vi "Master_DAQ_ReadVIN.vi"() -> (0 "cRIO Data":T1)   [LabVIEW 2017]
uses:
  TypeDef_cRIOData.ctl
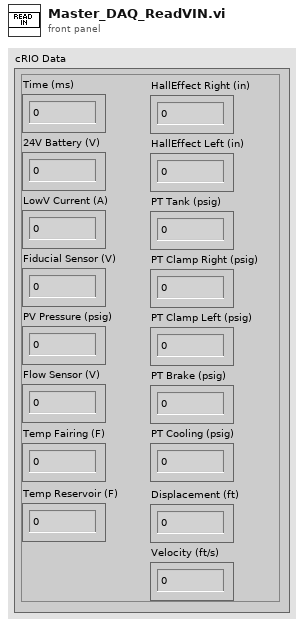
[diagram p1: front panel]
types:
  T1 = typedef "TypeDef_cRIOData.ctl" = cluster{"Time (ms)":dbl, "24V Battery (V)":dbl, "LowV Current (A)":dbl, "Fiducial Sensor (V)":dbl, "PV Pressure (psig)":dbl, "Flow Sensor (V)":dbl, "Temp Fairing (F)":dbl, "Temp Reservoir (F)":dbl, "HallEffect Right (in)":dbl, "HallEffect Left (in)":dbl, "PT Tank (psig)":dbl, "PT Clamp Right (psig)":dbl, "PT Clamp Left (psig)":dbl, "PT Brake (psig)":dbl, "PT Cooling (psig)":dbl, "Displacement (ft)":dbl, "Velocity (ft/s)":dbl}
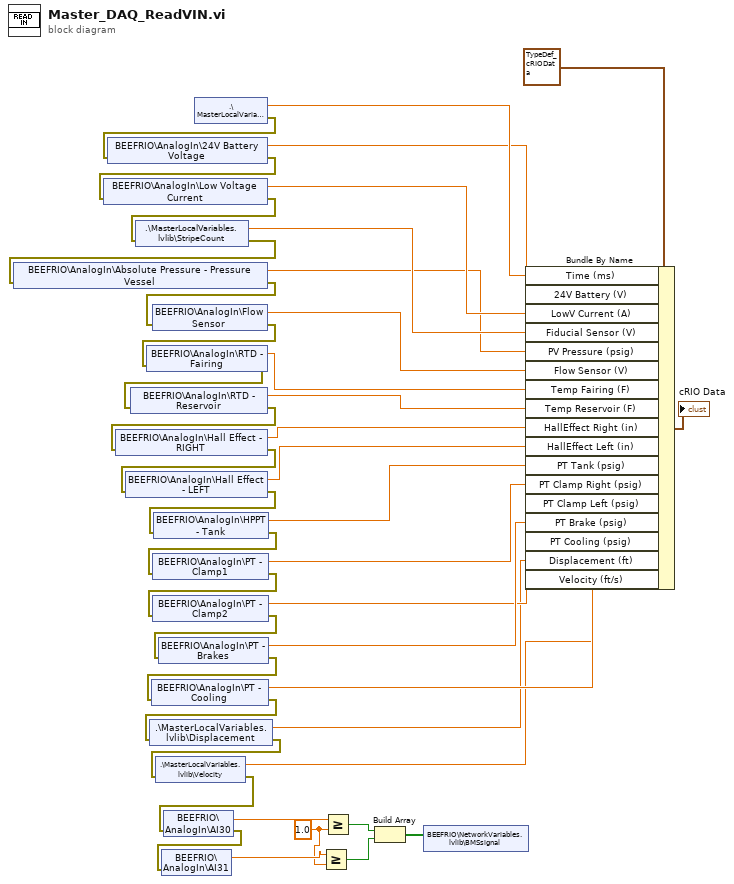
[diagram p0: block diagram]
diagram:
  w4 = 1.0 ("y")
  n1 = shared-variable ".\\MasterLocalVariables.lvlib\\Time"() -> (w41:dbl, error out=w40:errorcluster)  [unwired: 1 in]
  n2 = shared-variable "BEEFRIO\\AnalogIn\\24V Battery Voltage"(error in=w40) -> (w26:dbl, error out=w39:errorcluster)
  n3 = shared-variable "BEEFRIO\\AnalogIn\\Low Voltage Current"(error in=w39) -> (w25:dbl, error out=w38:errorcluster)
  n4 = shared-variable ".\\MasterLocalVariables.lvlib\\StripeCount"(error in=w38) -> (w24:dbl, error out=w37:errorcluster)
  n5 = shared-variable "BEEFRIO\\AnalogIn\\Absolute Pressure - Pressure Vessel"(error in=w37) -> (w23:dbl, error out=w36:errorcluster)
  n6 = shared-variable "BEEFRIO\\AnalogIn\\Flow Sensor"(error in=w36) -> (w22:dbl, error out=w35:errorcluster)
  n7 = shared-variable "BEEFRIO\\AnalogIn\\RTD - Fairing"(error in=w35) -> (w21:dbl, error out=w34:errorcluster)
  n8 = shared-variable "BEEFRIO\\AnalogIn\\RTD - Reservoir"(error in=w34) -> (w20:dbl, error out=w33:errorcluster)
  n9 = shared-variable "BEEFRIO\\AnalogIn\\Hall Effect - RIGHT"(error in=w33) -> (w19:dbl, error out=w32:errorcluster)
  n10 = shared-variable "BEEFRIO\\AnalogIn\\Hall Effect - LEFT"(error in=w32) -> (w18:dbl, error out=w27:errorcluster)
  n11 = shared-variable "BEEFRIO\\AnalogIn\\HPPT - Tank"(error in=w27) -> (w17:dbl, error out=w31:errorcluster)
  n12 = shared-variable "BEEFRIO\\AnalogIn\\PT - Clamp1"(error in=w31) -> (w13:dbl, error out=w30:errorcluster)
  n13 = shared-variable "BEEFRIO\\AnalogIn\\PT - Clamp2"(error in=w30) -> (w14:dbl, error out=w29:errorcluster)
  n14 = shared-variable "BEEFRIO\\AnalogIn\\PT - Brakes"(error in=w29) -> (w15:dbl, error out=w28:errorcluster)
  n15 = shared-variable "BEEFRIO\\AnalogIn\\PT - Cooling"(error in=w28) -> (w16:dbl, error out=w12:errorcluster)
  n16 = shared-variable ".\\MasterLocalVariables.lvlib\\Displacement"(error in=w12) -> (w10:dbl, error out=w11:errorcluster)
  n17 = shared-variable ".\\MasterLocalVariables.lvlib\\Velocity"(error in=w11) -> (w9:dbl, error out=w8:errorcluster)
  n18 = shared-variable "BEEFRIO\\AnalogIn\\AI30"(error in=w8) -> (w6:dbl, error out=w7:errorcluster)
  n19 = shared-variable "BEEFRIO\\AnalogIn\\AI31"(error in=w7) -> (w5:dbl)  [unwired: 1 out]
  n20 = Greater Or Equal?(x=w5, y=w4) -> (x >= y?=w3:bool)
  n21 = Greater Or Equal?(x=w6, y=w4) -> (x >= y?=w2:bool)
  n22 = Build Array(w2, w3) -> (w1:bool[])
  n23 = shared-variable "BEEFRIO\\NetworkVariables.lvlib\\BMSsignal"(w1) -> ()  [unwired: 1 in, 1 out]
  n24 = Bundle By Name(cluster=T1 {"Time (ms)"=0.0, "24V Battery (V)"=0.0, "LowV Current (A)"=0.0, "Fiducial Sensor (V)"=0.0, "PV Pressure (psig)"=0.0, "Flow Sensor (V)"=0.0, "Temp Fairing (F)"=0.0, "Temp Reservoir (F)"=0.0, "HallEffect Right (in)"=0.0, "HallEffect Left (in)"=0.0, "PT Tank (psig)"=0.0, "PT Clamp Right (psig)"=0.0, "PT Clamp Left (psig)"=0.0, "PT Brake (psig)"=0.0, "PT Cooling (psig)"=0.0, "Displacement (ft)"=0.0, "Velocity (ft/s)"=0.0} ("cRIO Data"), "Time (ms)"=w41, "24V Battery (V)"=w26, "LowV Current (A)"=w25, "Fiducial Sensor (V)"=w24, "PV Pressure (psig)"=w23, "Flow Sensor (V)"=w22, "Temp Fairing (F)"=w21, "Temp Reservoir (F)"=w20, "HallEffect Right (in)"=w19, "HallEffect Left (in)"=w18, "PT Tank (psig)"=w17, "PT Clamp Right (psig)"=w13, "PT Clamp Left (psig)"=w14, "PT Brake (psig)"=w15, "PT Cooling (psig)"=w16, "Displacement (ft)"=w10, "Velocity (ft/s)"=w9) -> (→"cRIO Data":T1)
